vi "HAPS_LoadTable_SetBeam_Manual.vi"() -> ()   [LabVIEW 2023, in "HAPS.lvlib"]
uses:
  HAPS.lvlib
  set_ele.ctl
  HAPS_SerialPort.ctl
  HAPS_MCU_ELE_Func.ctl
  <vilib>/Utility/file.llb/Read Delimited Spreadsheet (string).vi
panel:
  in  "set_ele":T1
  in  "file path (dialog if empty)":path
  in  "VISA resource name":refnum<visa-resource-name>="COM1"
  out "Remaining quantity":i32
  out "ele phase":i32
  out "ele gain":i32
  out "channel":i32
  out "chain ID":i32
  out "group":i32
  out "array id":i32
  # "HAPS 24x24 Setting\nManual In-Phase"
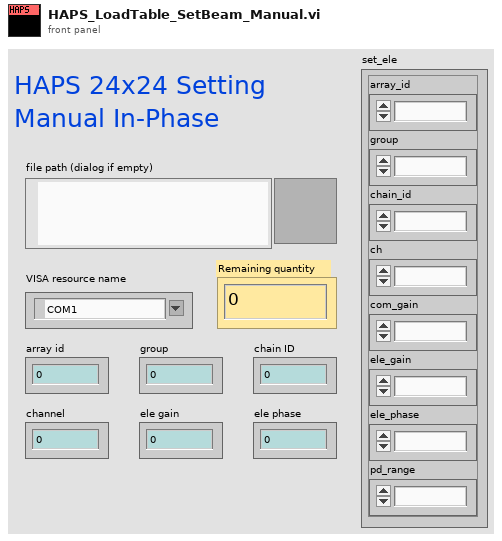
[diagram p1: front panel]
types:
  T1 = typedef "HAPS.lvlib/set_ele.ctl" = cluster{"ch":i32, "chain_id":i32, "group":i32, "array_id":i32, "ele_phase":i32, "ele_gain":i32, "com_gain":i32, "pd_range":i32}
  T2 = typedef "HAPS.lvlib/HAPS_SerialPort.ctl" = enum16{"Init", "Close", "CMD", "Flush"}
  T3 = typedef "HAPS.lvlib/HAPS_MCU_ELE_Func.ctl" = enum16{"array_init", "set_com_gain", "set_ch_gain_phase", "set_pd_range", "get_preamp_temp", "get_bfic_temp", "get_tx_pd", "ch_on", "ch_on_2", "ch_ctrl_all", "array_ctrl_src"}
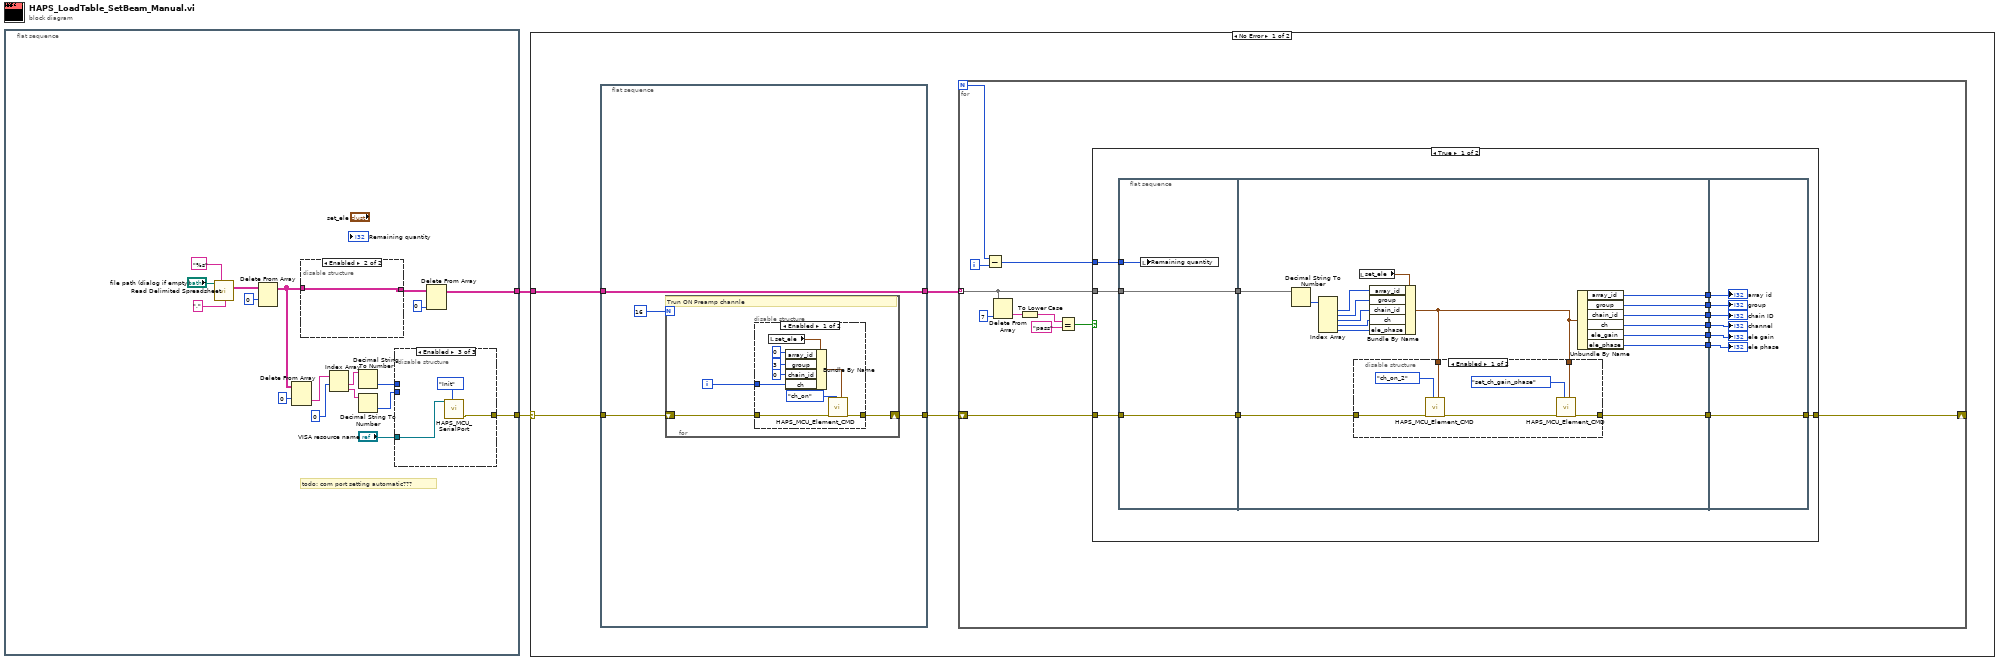
[diagram p0: block diagram]
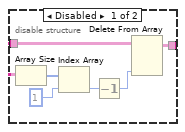
[diagram p2: hidden frame]
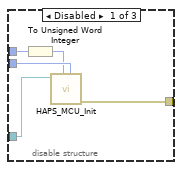
[diagram p3: hidden frame]
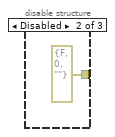
[diagram p4: hidden frame]
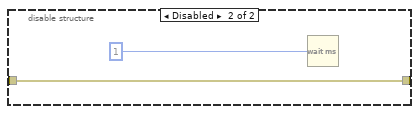
[diagram p6: hidden frame]
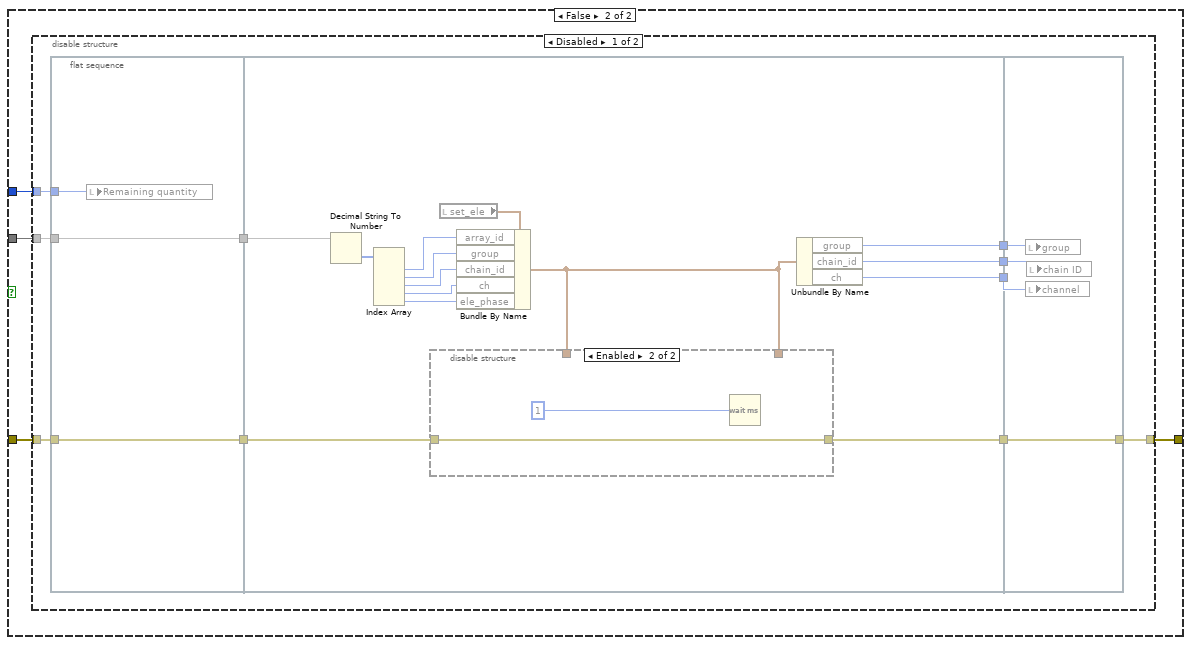
[diagram p7: hidden frame]
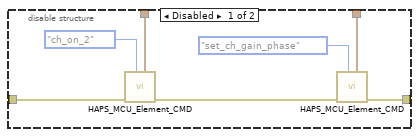
[diagram p8: hidden frame]
diagram:
  n1 = flat-sequence {
    tunnel: [w16] -> w2
    tunnel: [w14] -> w1
    frame #0 {
      # "todo: com port setting automatic???"
      n2 = call-poly <vilib>:"Read Delimited Spreadsheet.vi"("file path (dialog if empty)"="file path (dialog if empty)", "format (%s)"="%s" ("format (%.3f)"), "delimiter (\\t)"="," ("delimiter (\\t)")) -> ("all rows"=w18:string[][])  [unwired: 7 in, 5 out]
      n3 = Delete From Array(array=w18, index (row)=0) -> (array with subset deleted=w11:string[][])  [unwired: 2 in, 1 out]
      n4 = Delete From Array(array=w11, index (row)=0) -> (deleted portion=w10:string[])  [unwired: 2 in, 1 out]
      n5 = disable-structure shown="Enabled" {
        disable-tunnel: [w22 w27] -> w15
        disable-tunnel: w11 -> [w21 w27]
        frame Disabled {
          n6 = Array Size(array=w21) -> (size(s)=w26:i32[])
          n7 = Index Array(array=w26, index=1) -> (element=w23:i32)
          n8 = Decrement(x=w23) -> (x-1=w25:i32)
          n9 = Delete From Array(array=w21, index (col)=w25) -> (array with subset deleted=w22:string[][])  [unwired: 2 in, 1 out]
        }
        frame Enabled {
        }
      }
      n10 = Index Array(array=w10, index #1=0 ("index")) -> (element #1=w9:string, element #2=w8:string)  [unwired: 1 in]
      n11 = Decimal String To Number(string=w9) -> (number=w5:i32)  [unwired: 2 in, 1 out]
      n12 = Decimal String To Number(string=w8) -> (number=w4:i32)  [unwired: 2 in, 1 out]
      n13 = disable-structure shown="Enabled" {
        disable-tunnel: [w32 errorcluster {"status"=FALSE, "code"=0, "source"=""} ("error out") w36] -> w16
        disable-tunnel: w5 -> [w31 _ _]
        disable-tunnel: w4 -> [w30 _ _]
        disable-tunnel: "VISA resource name" -> [w29 _ w35]
        frame Disabled {
          n14 = To Unsigned Word Integer(number=w31) -> (unsigned 16bit integer=w28:u16)
          n15 = call "HAPS_MCU_Init.vi"("array_id"=w30, "Tx/Rx"=w28, "VISA resource name"=w29) -> ("error out"=w32:errorcluster)  [unwired: 8 in]
        }
        frame Disabled {
        }
        frame Enabled {
          n16 = call "HAPS_MCU_SerialPort.vi"("HAPS_SerialPort_Func"=HAPS_SerialPort."Init", "VISA resource name"=w35) -> ("error out"=w36:errorcluster)  [unwired: 7 in, 2 out]
        }
      }
      n17 = Delete From Array(array=w15, index (col)=0 ("index (row)")) -> (array with subset deleted=w14:string[][])  [unwired: 2 in, 1 out]
    }
  }
  n18 = case shown="No Error" w2 {
    selector: w2 -> [w40 _]
    tunnel: w1 -> [w39 _]
    frame No Error {
      n19 = flat-sequence {
        tunnel: w40 -> [w42]
        tunnel: w39 -> [w44]
        tunnel: [w44] -> w38
        tunnel: [w43] -> w37
        frame #0 {
          n20 = for {
            N: 16 -> [_]
            shift-right: [w47] -> w43
            shift-left: w42 -> [w46]
            i -> [w45]
            # "Trun ON Preamp channle"
            n21 = disable-structure shown="Enabled" {
              disable-tunnel: [w56 w57] -> w47
              disable-tunnel: w46 -> [w55 w57]
              disable-tunnel: w45 -> [w50 _]
              frame Enabled {
                n22 = local read "set_ele"() -> (w54:T1)
                n23 = Bundle By Name(cluster=w54, "array_id"=0, "group"=3, "chain_id"=0, "ch"=w50) -> (w53:T1)
                n24 = call "HAPS_MCU_Element_CMD.vi"("set_ele"=w53, "HAPS_MCU_ELE_Func."=HAPS_MCU_ELE_Func."ch_on", "error in"=w55) -> ("error out"=w56:errorcluster)  [unwired: 7 in, 1 out]
              }
              frame Disabled {
              }
            }
          }
        }
      }
      n25 = for {
        N -> [w65]
        tunnel: w38 -> [w63] mode=indexing
        shift-right: [w68] -> _
        shift-left: w37 -> [w67]
        i -> [w66]
        n26 = Subtract(x=w65, y=w66) -> (x-y=w64:i32)
        n27 = Delete From Array(array=w63, index=7) -> (deleted portion=w61:string)  [unwired: 1 in, 1 out]
        n28 = To Lower Case(string=w61) -> (all lower case string=w60:string)
        n29 = Equal?(x=w60, y="pass") -> (x = y?=w58:bool)
        n30 = case shown="True" w58 {
          tunnel: [w72 w121] -> w68
          tunnel: w67 -> [w71 w120]
          tunnel: w64 -> [w70 w119]
          tunnel: w63 -> [w69 w118]
          frame True {
            n31 = flat-sequence {
              tunnel: w71 -> [w83]
              tunnel: w69 -> [w84]
              tunnel: [w84] -> w81
              tunnel: [w83] -> w80
              tunnel: w70 -> [w82]
              tunnel: w81 -> [w101]
              tunnel: w80 -> [w98]
              tunnel: [w99] -> w79
              tunnel: [w92] -> w78
              tunnel: [w91] -> w77
              tunnel: [w90] -> w76
              tunnel: [w89] -> w75
              tunnel: [w88] -> w74
              tunnel: [w87] -> w73
              tunnel: [w117] -> w72
              tunnel: w79 -> [w117]
              tunnel: w78 -> [w116]
              tunnel: w77 -> [w115]
              tunnel: w76 -> [w114]
              tunnel: w75 -> [w113]
              tunnel: w74 -> [w112]
              tunnel: w73 -> [w111]
              frame #0 {
                n32 = local write "Remaining quantity"(w82) -> ()
              }
              frame #1 {
                n33 = Decimal String To Number(string=w101) -> (number=w100:i32[])  [unwired: 2 in, 1 out]
                n34 = Index Array(array=w100) -> (element #1=w97:i32, element #2=w96:i32, element #3=w95:i32, element #4=w94:i32, element #5=w93:i32)  [unwired: 5 in]
                n35 = local read "set_ele"() -> (w85:T1)
                n36 = Bundle By Name(cluster=w85, "array_id"=w97, "group"=w96, "chain_id"=w95, "ch"=w94, "ele_phase"=w93) -> (w86:T1)
                n37 = disable-structure shown="Enabled" {
                  disable-tunnel: [w108 w110] -> w99
                  disable-tunnel: w98 -> [w102 w110]
                  disable-tunnel: w86 -> [w106 _]
                  disable-tunnel: w86 -> [w105 _]
                  frame Enabled {
                    n38 = call "HAPS_MCU_Element_CMD.vi"("set_ele"=w105, "HAPS_MCU_ELE_Func."=HAPS_MCU_ELE_Func."ch_on_2", "error in"=w102) -> ("error out"=w103:errorcluster)  [unwired: 7 in, 1 out]
                    n39 = call "HAPS_MCU_Element_CMD.vi"("set_ele"=w106, "HAPS_MCU_ELE_Func."=HAPS_MCU_ELE_Func."set_ch_gain_phase", "error in"=w103) -> ("error out"=w108:errorcluster)  [unwired: 7 in, 1 out]
                  }
                  frame Disabled {
                    n40 = Wait (ms)(milliseconds to wait=u32 1) -> ()  [unwired: 1 out]
                  }
                }
                n41 = Unbundle By Name(w86) -> ("array_id"=w92:i32, "group"=w91:i32, "chain_id"=w90:i32, "ch"=w89:i32, "ele_gain"=w88:i32, "ele_phase"=w87:i32)
              }
              frame #2 {
                "group" <- w115
                "chain ID" <- w114
                "channel" <- w113
                "ele gain" <- w112
                "ele phase" <- w111
                "array id" <- w116
              }
            }
          }
          frame False {
            n42 = disable-structure shown="Disabled" {
              disable-tunnel: [w125 _] -> w121
              disable-tunnel: w120 -> [w124 _]
              disable-tunnel: w119 -> [w123 _]
              disable-tunnel: w118 -> [w122 _]
              frame Disabled {
                n43 = flat-sequence {
                  tunnel: w124 -> [w133]
                  tunnel: w122 -> [w134]
                  tunnel: [w134] -> w131
                  tunnel: [w133] -> w130
                  tunnel: w123 -> [w132]
                  tunnel: w131 -> [w148]
                  tunnel: w130 -> [w145]
                  tunnel: [w146] -> w129
                  tunnel: [w139] -> w128
                  tunnel: [w138] -> w127
                  tunnel: [w135] -> w126
                  tunnel: [w161] -> w125
                  tunnel: w129 -> [w161]
                  tunnel: w128 -> [w160]
                  tunnel: w127 -> [w159]
                  tunnel: w126 -> [w158]
                  frame #0 {
                    n44 = local write "Remaining quantity"(w132) -> ()
                  }
                  frame #1 {
                    n45 = Decimal String To Number(string=w148) -> (number=w147:i32[])  [unwired: 2 in, 1 out]
                    n46 = Index Array(array=w147) -> (element #1=w144:i32, element #2=w143:i32, element #3=w142:i32, element #4=w141:i32, element #5=w140:i32)  [unwired: 5 in]
                    n47 = local read "set_ele"() -> (w136:T1)
                    n48 = Bundle By Name(cluster=w136, "array_id"=w144, "group"=w143, "chain_id"=w142, "ch"=w141, "ele_phase"=w140) -> (w137:T1)
                    n49 = disable-structure shown="Enabled" {
                      disable-tunnel: [w155 w157] -> w146
                      disable-tunnel: w145 -> [w149 w157]
                      disable-tunnel: w137 -> [w153 _]
                      disable-tunnel: w137 -> [w152 _]
                      frame Disabled {
                        n50 = call "HAPS_MCU_Element_CMD.vi"("set_ele"=w152, "HAPS_MCU_ELE_Func."=HAPS_MCU_ELE_Func."ch_on_2", "error in"=w149) -> ("error out"=w150:errorcluster)  [unwired: 7 in, 1 out]
                        n51 = call "HAPS_MCU_Element_CMD.vi"("set_ele"=w153, "HAPS_MCU_ELE_Func."=HAPS_MCU_ELE_Func."set_ch_gain_phase", "error in"=w150) -> ("error out"=w155:errorcluster)  [unwired: 7 in, 1 out]
                      }
                      frame Enabled {
                        n52 = Wait (ms)(milliseconds to wait=u32 1) -> ()  [unwired: 1 out]
                      }
                    }
                    n53 = Unbundle By Name(w137) -> ("group"=w139:i32, "chain_id"=w138:i32, "ch"=w135:i32)
                  }
                  frame #2 {
                    n54 = local write "group"(w160) -> ()
                    n55 = local write "channel"(w158) -> ()
                    n56 = local write "chain ID"(w159) -> ()
                  }
                }
              }
              frame Enabled {
              }
            }
          }
        }
      }
    }
    frame Error {
    }
  }
